vi "Write OutIndex.vi"(8 "error in (no error)":errorcluster, 10 "OutIndex":i32, 11 "Station Action in":refnum<class "Station Action.lvclass">) -> (0 "error out":errorcluster, 3 "Station Action out":refnum<class "Station Action.lvclass">)   [LabVIEW 2019, in "Station Action.lvclass"]
uses:
  Station Action.lvclass
  Station Action.lvclass/Station Action.ctl
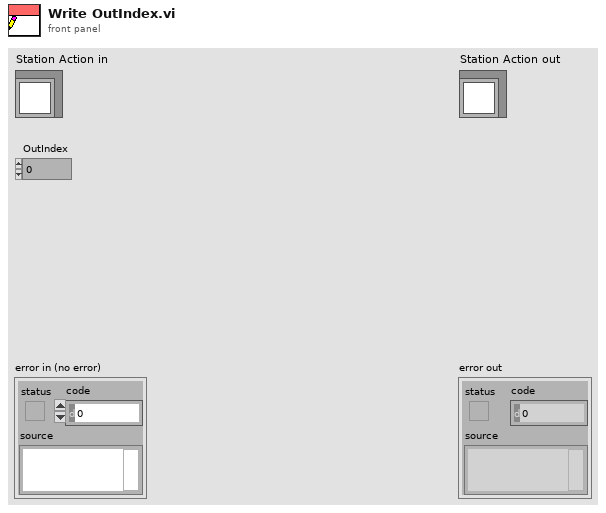
[diagram p1: front panel]
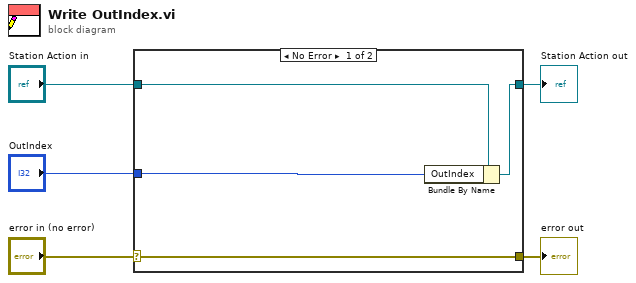
[diagram p0: block diagram]
diagram:
  n1 = case shown="No Error" "error in (no error)" {
    selector: "error in (no error)" -> [w9 w10]
    tunnel: [w9 w10] -> w4
    tunnel: [w7 w11] -> w2
    tunnel: "Station Action in" -> [w8 w11]
    tunnel: "OutIndex" -> [w6 _]
    frame No Error {
      n2 = Bundle By Name(cluster=w8, "OutIndex"=w6) -> (w7:refnum<class "Station Action.lvclass">)
    }
    frame Error {
    }
  }
  "error out" <- w4
  "Station Action out" <- w2
